vi "Render Window Open.vi"(6 "Control Ref Queue":T2, 8 "error in (no error)":errorcluster, 11 "Object Cluster In":T1) -> (0 "error out":errorcluster, 3 "Object Cluster Out":T1)   [LabVIEW 2020, in "3D Plot.lvclass"]
uses:
  3D Plot.lvclass
  3DMathPlot Ctrl Act Queue.ctl
  3DMathPlot Ctrl Act Cluster.ctl
  3DMathPlot State Class.ctl
  Object Cluster.ctl
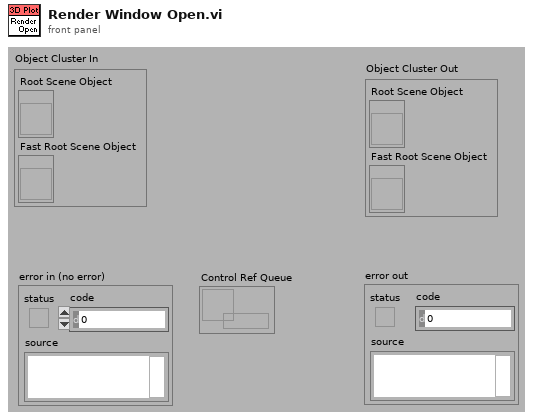
[diagram p1: front panel]
types:
  T1 = typedef "3D Plot.lvclass/Object Cluster.ctl" = cluster{"Root Scene Object":refnum<vi>, "Fast Root Scene Object":refnum<vi>}
  T2 = typedef "3DMathPlot Ctrl Act Queue.ctl" = refnum<queue>
  T3 = cluster{"Left":i16, "Top":i16, "Right":i16, "Bottom":i16}
  T4 = enum16{"Open", "Minimized", "Maximized", "Hidden"}
  T5 = typedef "3DMathPlot Ctrl Act Cluster.ctl" = cluster{"3D Picture Control":refnum<vi>, "Render Window Refnum":refnum<vi>, "XY Graph":refnum<vi>, "Intensity Graph":refnum<vi>, "Color Legend Palette":refnum<vi>, "Projection Palette":refnum<vi>, "XControl  Ref":refnum<vi>, "Facade Ref":refnum<vi>, "Export Image Ref":refnum<vi>, "Clear Data Flag":bool, "Display State Change Class":T6}
  T6 = typedef "3DMathPlot State Class.ctl" = enum16{"Update All Objects (Undo)", "Update Light Object Only", "Update Axis Object Only", "Update Plot Object Only", "Update Cursor Object Only", "Update Axis Plot Cursor Objects", "No Update"}
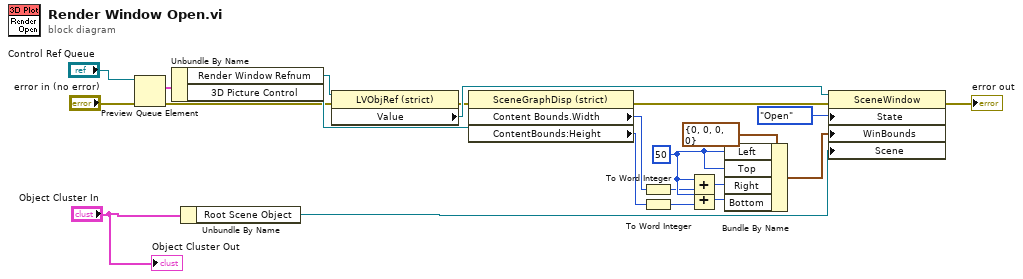
[diagram p0: block diagram]
diagram:
  w15 = i16 50
  n1 = Preview Queue Element(queue="Control Ref Queue", error in (no error)="error in (no error)") -> (element=w5:T5, error out=w4:errorcluster)  [unwired: 3 out]
  n2 = Unbundle By Name(w5) -> ("Render Window Refnum"=w6:refnum<vi>, "3D Picture Control"=w7:refnum<vi>)
  n3 = Unbundle By Name("Object Cluster In") -> ("Root Scene Object"=w1:refnum<vi>)
  n4 = property class="LVObjRef (strict)"(reference=w6, error in=w4) -> (error out=w9:errorcluster, "Value"=w10:refnum<vi>)  [unwired: 1 out]
  n5 = property on="Property Node" class="SceneGraphDisp (strict)"(reference=w7, error in=w9) -> (error out=w8:errorcluster, "Content Bounds.Width"=w17:u32, "ContentBounds:Height"=w18:u32)  [unwired: 1 out]
  n6 = To Word Integer(number=w17) -> (16bit integer=w3:i16)
  n7 = To Word Integer(number=w18) -> (16bit integer=w2:i16)
  n8 = Add(x=w15, y=w3) -> (x+y=w14:i16)
  n9 = Add(x=w15, y=w2) -> (x+y=w16:i16)
  n10 = Bundle By Name(cluster=T3 {"Left"=0, "Top"=0, "Right"=0, "Bottom"=0} ("Window Bounds"), "Left"=w15, "Top"=w15, "Right"=w14, "Bottom"=w16) -> (w13:T3)
  n11 = property class="SceneWindow"(reference=w10, error in=w8, "State"=T4."Open" ("Window State"), "WinBounds"=w13, "Scene"=w1) -> (error out=→"error out":errorcluster)  [unwired: 1 out]
  "Object Cluster Out" <- "Object Cluster In"
